vi "Make Window Always on Top.vi"(4 "error in (no error)":errorcluster, 5 "activate? (F)":bool, 6 "window name (\"\")":string, 7 "window refnum (NaWR)":T1) -> (0 "error out":errorcluster, 3 "window refnum out":T1)   [LabVIEW 2023, in "WINUTIL.lvlib"]
doc: "This function will make the window named in the 'window name' input, or identified by the 'window refnum' the topmost window, so it will always be on top of other windows. If 'not a window refnum' is passed in, then the function will use the window name to get a window window refnum. If the window cannot be found, an error will be returned."
uses:
  WINUTIL.lvlib
  Window Refnum.ctl
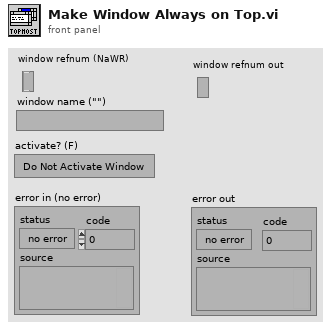
[diagram p1: front panel]
types:
  T1 = typedef "WINUTIL.lvlib/Window Refnum.ctl" = refnum<k1>
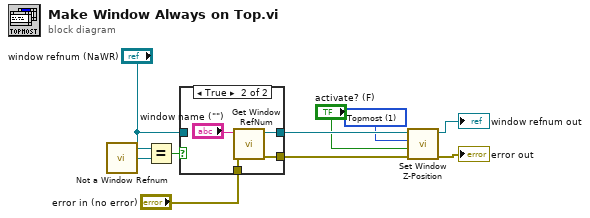
[diagram p0: block diagram]
diagram:
  w2 = i16 1 items=["Not Topmost", "Topmost", "Top", "Bottom"]
  n1 = call "Not a Window Refnum.vi"() -> ("Not a Window Refnum"=w8:T1)
  n2 = Equal?(x="window refnum (NaWR)", y=w8) -> (x = y?=w9:bool)
  n3 = case shown="True" w9 {
    tunnel: "error in (no error)" -> [w11 w16]
    tunnel: [w12 w15] -> w6
    tunnel: "window refnum (NaWR)" -> [w12 _]
    tunnel: [w11 w14] -> w5
    frame False {
    }
    frame True {
      n4 = call "Get Window RefNum.vi"("error in (no error)"=w16, "window name (\"\")"="window name (\"\")") -> ("error out"=w14:errorcluster, "window refnum (NaWR)"=w15:T1)  [unwired: 6 out]
    }
  }
  n5 = call "Set Window Z-Position.vi"("error in (no error)"=w5, "activate? (T)"="activate? (F)", "z-order position"=w2, "window refnum"=w6) -> ("error out"=→"error out":errorcluster, "window refnum out"=→"window refnum out":T1)  [unwired: 2 out]
